vi "PageDialog.vi"(10 "Nr of Pages":u16) -> (2 "OpenPage..":u16)   [LabVIEW 2014, in "LAVA TIFF File Reader.lvlib"]
uses:
  LAVA TIFF File Reader.lvlib
panel:
  in  "OK Button":bool
  in  "Page":u16 min=1 max=3
  # "There are"
  # "Open Page Nr."
  # "in the Document"
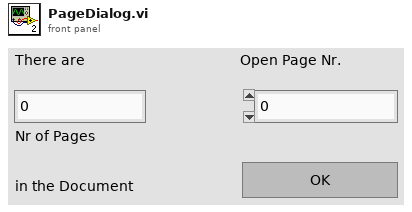
[diagram p1: front panel]
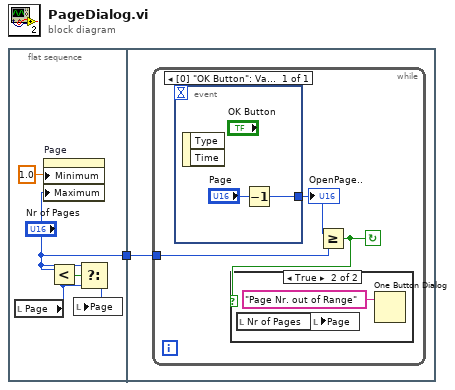
[diagram p0: block diagram]
diagram:
  n1 = flat-sequence {
    tunnel: ["Nr of Pages"] -> w1
    tunnel: w1 -> [w7]
    frame #0 {
      n2 = local read "Page"() -> (w3:u16)
      n3 = property on="Page" class="DigNum (strict)"("Minimum"=1.0 ("Data Entry Limits:Minimum"), "Maximum"="Nr of Pages") -> ()  [unwired: 2 in, 2 out]
      n4 = Less?(x="Nr of Pages", y=w3) -> (x < y?=w5:bool)
      n5 = Select(t="Nr of Pages", s=w5, f=w3) -> (s? t:f=w2:u16)
      n6 = local write "Page"(w2) -> ()
    }
    frame #1 {
      n7 = while {
        tunnel: w7 -> [w9]
        stop <- w8 continue-if-true
        n8 = event shown="[0] \"OK Button\": Value Change;  Panel Close" {
          selector: _ -> [_]
          dyn-events: _ -> [_]
          timeout: _ -> [_]
          tunnel: [w13] -> w10
          event "OK Button": Value Change; Panel Close {
            n9 = event-data() -> ()  [unwired: 1 in, 2 out]
            n10 = Decrement(x="Page") -> (x-1=w13:u16)
          }
        }
        "OpenPage.." <- w10
        n11 = Greater Or Equal?(x=w10, y=w9) -> (x >= y?=w8:bool)
        n12 = case shown="True" w8 {
          frame False {
          }
          frame True {
            n13 = local read "Nr of Pages"() -> (w11:u16)
            n14 = local write "Page"(w11) -> ()
            n15 = One Button Dialog(message="Page Nr. out of Range") -> ()  [unwired: 1 in, 1 out]
          }
        }
      }
    }
  }
